vi "Read Counter.vi"(8 "error in (no error)":errorcluster, 11 "Connection Data In":T1) -> (0 "error out":errorcluster, 2 "CounterValue":u64, 3 "Connection Data Out":T1)   [LabVIEW 2014, in "MSX-E3711_dll.lvlib"]
uses:
  MSX-E3711_dll.lvlib
  Typedef/Connection Data.ctl
  E:/Repositorio Magnis/INF002/v0/Modules/HAL/Drivers/Sync/ADDI-DATA MSX-E3711/API/MSXE371x.dll
  MSXE371x.dll
  E:/Repositorio Magnis/INF002/v0/Modules/HAL/Drivers/Sync/ADDI-DATA MSX-E3711/API/MXCommon.dll
  MXCommon.dll
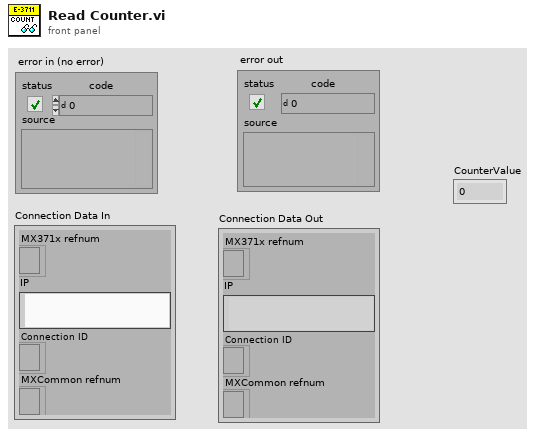
[diagram p1: front panel]
types:
  T1 = typedef "MSX-E3711_dll.lvlib/Connection Data.ctl" = cluster{"MX371x refnum":refnum<k24>, "IP":string, "Connection ID ":refnum<k5>, "MXCommon refnum":refnum<k24>}
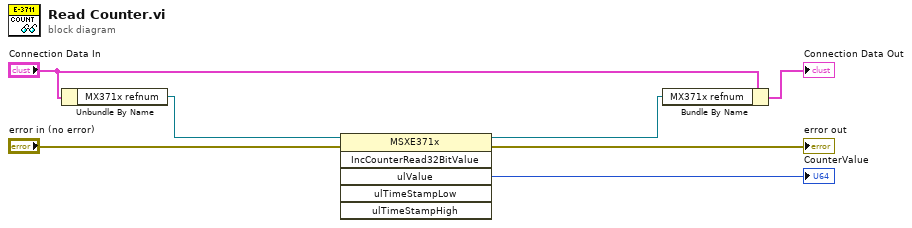
[diagram p0: block diagram]
diagram:
  n1 = Unbundle By Name("Connection Data In") -> ("MX371x refnum"=w5:refnum<k24>)
  n2 = invoke class="MSXE371x" method="IncCounterRead32BitValue"(reference=w5, error in="error in (no error)") -> (reference out=w2:refnum<k24>, error out=→"error out":errorcluster, "ulValue"=→"CounterValue":u64)  [unwired: 4 in, 3 out]
  n3 = Bundle By Name(cluster="Connection Data In", "MX371x refnum"=w2) -> (→"Connection Data Out":T1)
